vi "Close My Data HDF5.vi"(8 "error in":errorcluster, 11 "file refnum":T1) -> (0 "error out":errorcluster)   [LabVIEW 2014]
uses:
  My Data HDF5 Refs.ctl
  <vilib>/UPVI/lvhdf5/library.llb/HDF5 Ref.ctl
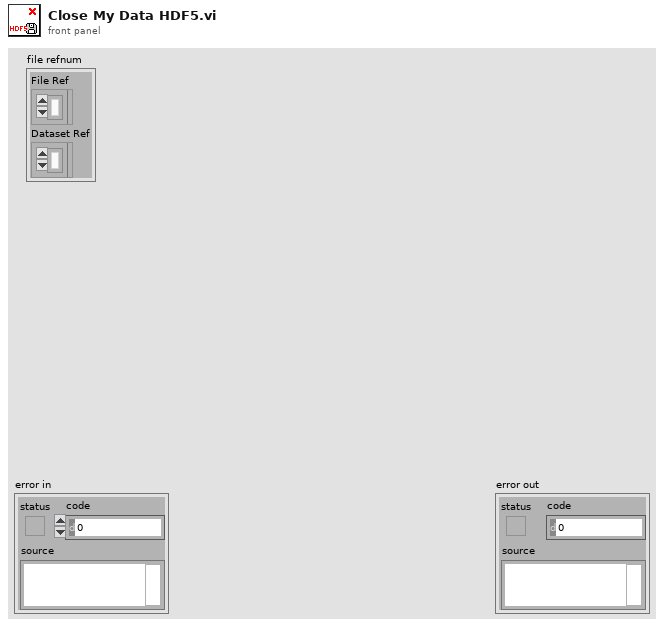
[diagram p1: front panel]
types:
  T1 = typedef "My Data HDF5 Refs.ctl" = cluster{"File Ref":T2, "Dataset Ref":T2}
  T2 = typedef "HDF5 Ref.ctl" = refnum<k1>
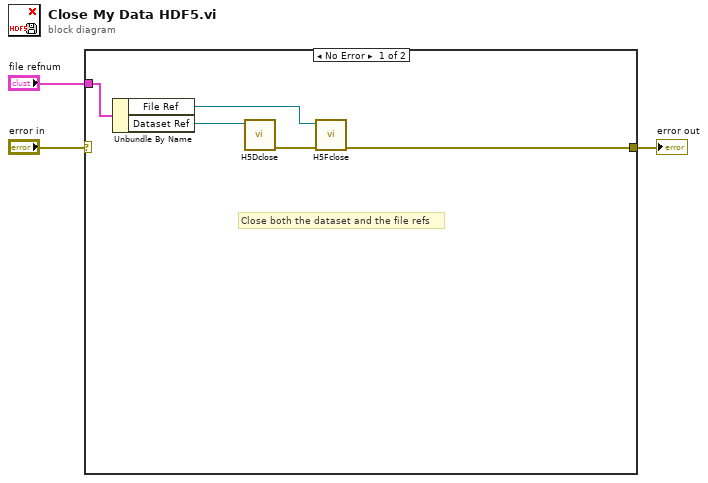
[diagram p0: block diagram]
diagram:
  n1 = case shown="No Error" "error in" {
    selector: "error in" -> [_ w9]
    tunnel: [w4 w9] -> w3
    tunnel: "file refnum" -> [w8 _]
    frame No Error {
      # "Close both the dataset and the file refs"
      n2 = Unbundle By Name(w8) -> ("File Ref"=w5:T2, "Dataset Ref"=w7:T2)
      n3 = call <vilib>:"H5Dclose.vi"("HDF5 Dataset Ref"=w7) -> ("error out"=w6:errorcluster)  [unwired: 8 in]
      n4 = call <vilib>:"H5Fclose.vi"("error in (no error)"=w6, "HDF5 Ref"=w5) -> ("error out"=w4:errorcluster)  [unwired: 7 in]
    }
    frame Error {
      # "Wire previous error through"
    }
  }
  "error out" <- w3
